vi "Convert from JSON Comp Format.vi"(8 "error in (no error)":errorcluster, 11 "JSON format":T2) -> (0 "error out":errorcluster, 3 "digital audio protocol settings":T1)   [LabVIEW 2021, in "digital audio protocol controls.lvlib"]
uses:
  digital audio protocol controls.lvlib
  digital audio protocol settings_json.ctl
  digital audio protocol settings.ctl
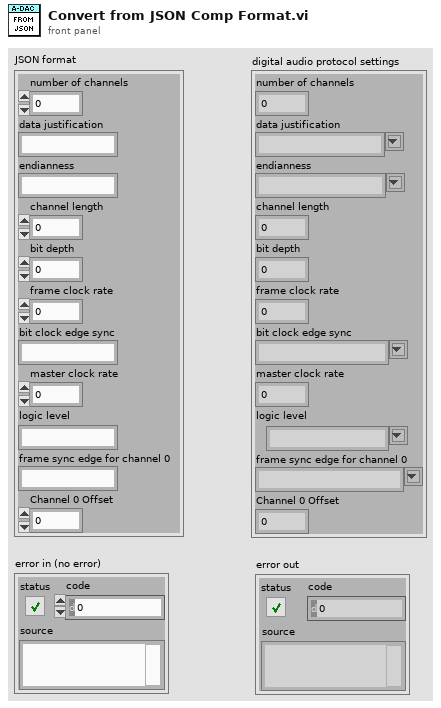
[diagram p1: front panel]
types:
  T1 = typedef "digital audio protocol controls.lvlib/digital audio protocol settings.ctl" = cluster{"number of channels":u32, "data justification":string, "endianness":string, "channel length":u32, "bit depth":u32, "frame clock rate":dbl, "bit clock edge sync":string, "master clock rate":dbl, "logic level":string, "frame sync edge for channel 0":string, "Channel 0 Offset":u32}
  T2 = typedef "digital audio protocol controls.lvlib/digital audio protocol settings_json.ctl" = cluster{"number of channels":u32, "data justification":string, "endianness":string, "channel length":u32, "bit depth":u32, "frame clock rate":dbl, "bit clock edge sync":string, "master clock rate":dbl, "logic level":string, "frame sync edge for channel 0":string, "Channel 0 Offset":u32}
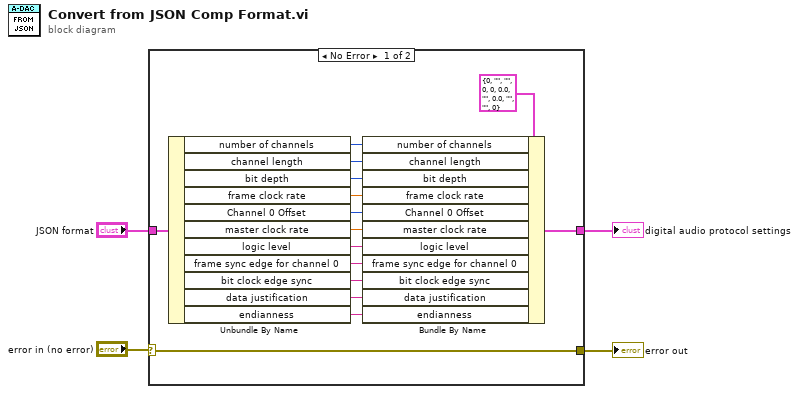
[diagram p0: block diagram]
diagram:
  n1 = case shown="No Error" "error in (no error)" {
    selector: "error in (no error)" -> [w5 w20]
    tunnel: "JSON format" -> [w13 _]
    tunnel: [w12 _] -> w3
    tunnel: [w5 w20] -> w1
    frame No Error {
      n2 = Unbundle By Name(w13) -> ("number of channels"=w19:u32, "channel length"=w18:u32, "bit depth"=w17:u32, "frame clock rate"=w16:dbl, "Channel 0 Offset"=w11:u32, "master clock rate"=w15:dbl, "logic level"=w10:string, "frame sync edge for channel 0"=w9:string, "bit clock edge sync"=w8:string, "data justification"=w7:string, "endianness"=w6:string)
      n3 = Bundle By Name(cluster=T1 {"number of channels"=0, "data justification"="", "endianness"="", "channel length"=0, "bit depth"=0, "frame clock rate"=0.0, "bit clock edge sync"="", "master clock rate"=0.0, "logic level"="", "frame sync edge for channel 0"="", "Channel 0 Offset"=0} ("digital audio protocol settings"), "number of channels"=w19, "channel length"=w18, "bit depth"=w17, "frame clock rate"=w16, "Channel 0 Offset"=w11, "master clock rate"=w15, "logic level"=w10, "frame sync edge for channel 0"=w9, "bit clock edge sync"=w8, "data justification"=w7, "endianness"=w6) -> (w12:T1)
    }
    frame Error {
    }
  }
  "digital audio protocol settings" <- w3
  "error out" <- w1
